vi "ATF Storage-DO_Write.vi"(7 "Period":i64=100, 8 "error in (no error)":errorcluster, 10 "Data FIFO Ref":T1, 11 "Refnum in":refnum<k21>) -> (0 "error out":errorcluster, 3 "Refnum out":refnum<k21>)   [LabVIEW 2022 SP3]
uses:
  RT Controls/ATF Storage-Data FIFO.ctl
  <vilib>/Platform/TimedLoop/XDataNode/timing_clust.ctl
  <vilib>/Platform/TimedLoop/XDataNode/nitl_modes.ctl
  <vilib>/Platform/TimedLoop/XDataNode/wakeup.ctl
  RT Controls/ATF Storage Haelth.ctl
  <vilib>/DAQmx/write.llb/DAQmx Write (Digital 1D Bool NChan 1Samp 1Line).vi
  RT Support/ATF Storage-RT_Global_R.vi
  <vilib>/DAQmx/miscellaneous.llb/DAQmx Fill In Error Info.vi
  <vilib>/platform/TimedLoop/XDataNode/XDataNode.xnode
  <vilib>/Platform/TimedLoop/XDataNode/XDNodeRunTimeDep.lvlib
panel:
  out "overflow?":bool
  out "x":u32
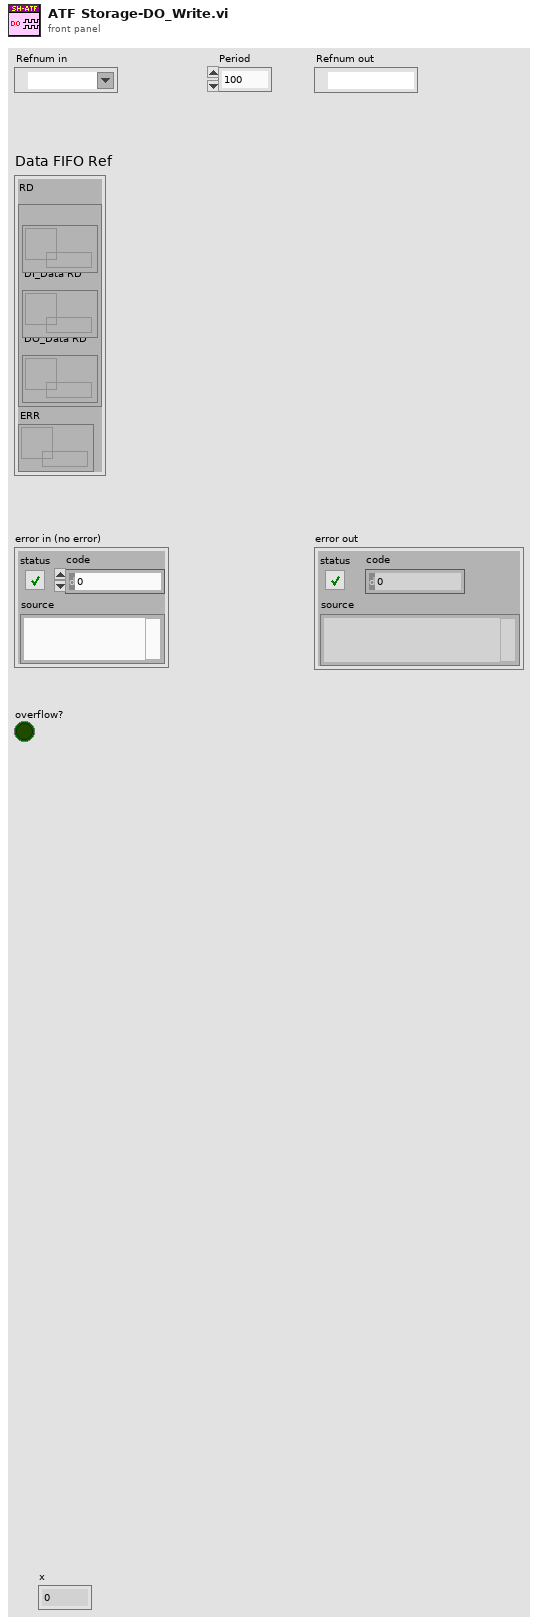
[diagram p1: front panel]
types:
  T1 = typedef "ATF Storage-Data FIFO.ctl" = cluster{"RD":cluster{"AI_V_Data RD":refnum<queue>, "DI_Data RD":refnum<queue>, "DO_Data RD":refnum<queue>}, "ERR":refnum<queue>}
  T2 = enum16{"Init", "Read", "Write 'All'", "Write 'n'", "Write Safe Value", "Write Start Time", "Overwrite Pattern", "Overwrite Pattern with Start", "Append Pattern", "Start Pattern Mode", "Abort Pattern Mode", "Read 1"}
  T3 = typedef "XDNodeRunTimeDep.lvlib/timing_clust.ctl" = cluster{"Expected End [f-1]":u64, "Actual End [f-1]":u64, "Finished Late? [f-1]":bool, "Expected End [i-1]":u64, "Actual End [i-1]":u64, "Finished Late? [i-1]":bool, "Expected Start [i]":u64, "Actual Start [i]":u64, "Expected Start [f]":u64, "Actual Start [f]":u64, "Source Name":string, "Structure Name":string, "Period":i64, "Deadline":i64, "Offset":i64, "Start":i64, "Priority":i32, "Timeout":i32, "Mode":T4, "Wakeup Reason":T5, "Error":errorcluster, "Source Type":string, "Secondary Source Type":string, "Global End Time":u64, "Global Start Time":u64, "Frame Duration":u64, "Iteration Duration":u64, "Assigned CPU":i32, "I/O Scan Engine Mode":u32}
  T4 = typedef "XDNodeRunTimeDep.lvlib/nitl_modes.ctl" = enum32{"No Change", "Process missed periods, maintain original phase", "Discard missed periods, maintain original phase", "Process missed periods, ignore original phase", "Discard missed periods, ignore original phase"}
  T5 = typedef "XDNodeRunTimeDep.lvlib/wakeup.ctl" = enum32{"Normal", "Aborted", "Asynchronous wakeup", "Timing source error", "Timed loop error", "Timeout"}
  T6 = typedef "ATF Storage Haelth.ctl" = enum16{"AI C", "AI V", "AO", "DI", "DO", "TC", "ACC", "RT Str", "DR A"}
  T7 = enum16{"Init", "Read 'All'", "Read 'n'", "Read '1'", "Write '1'", "Write 'n'", "Write 'All'"}
  T8 = cluster{"Start DAQ":bool, "Stop DAQ":bool, "RT Stop":bool, "RT Exit":bool, "Start Seq":bool}
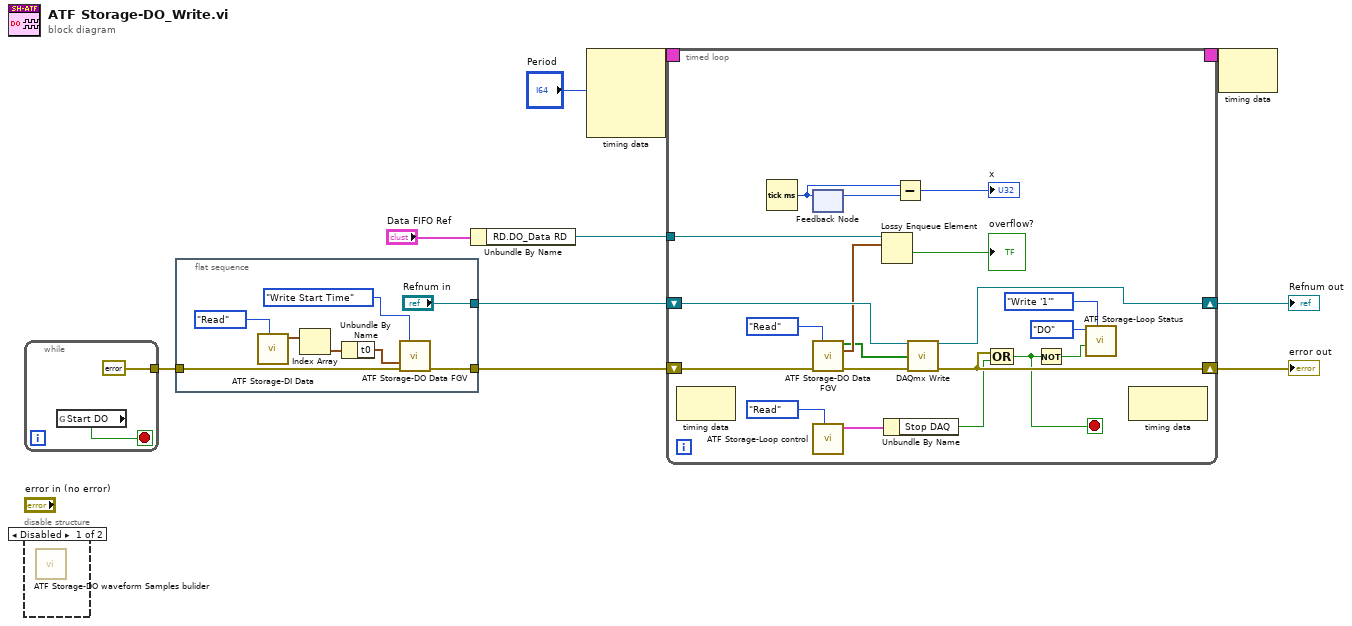
[diagram p0: block diagram]
diagram:
  n1 = while {
    tunnel: [errorcluster {"status"=FALSE, "code"=0, "source"=""} ("error in (no error)")] -> w4
    stop <- w12 stop-if-true
    n2 = global read "ATF Storage-RT_Global_R.vi" "Start DO"() -> (w12:bool)
  }
  n3 = disable-structure shown="Disabled" {
    frame Disabled {
      n4 = call "ATF Storage-DO waveform Samples bulider.vi"() -> ()  [unwired: 12 in]
    }
    frame Enabled {
    }
  }
  n5 = flat-sequence {
    tunnel: w4 -> [w18]
    tunnel: ["Refnum in"] -> w6
    tunnel: [w19] -> w5
    frame #0 {
      n6 = call "ATF Storage-DI Data.vi"("Enum"=enum16{"Write", "Read"}."Read") -> ("Out_DI data"=w17:digitalwaveform[])  [unwired: 10 in]
      n7 = Index Array(array=w17) -> (element=w16:digitalwaveform)  [unwired: 1 in]
      n8 = Unbundle By Name(w16) -> ("t0"=w14:timestamp)
      n9 = call "ATF Storage-DO Data FGV.vi"("Option"=T2."Write Start Time", "Time Stamp In"=w14, "error in (no error)"=w18) -> ("error out"=w19:errorcluster)  [unwired: 6 in, 6 out]
    }
  }
  n10 = Unbundle By Name("Data FIFO Ref") -> ("RD.DO_Data RD"=w7:refnum<queue>)
  n11 = node-c288("Period") -> (w3:T3)  [unwired: 3 in]
  n12 = timed-loop {
    tunnel: w7 -> [w37]
    shift-right: [w38] -> w9
    shift-left: w6 -> [w40]
    shift-right: [w39] -> w10
    shift-left: w5 -> [w30]
    timing: w3 -> [_]
    timing-out: [_] -> w2
    stop <- w21 stop-if-true
    n13 = node-c288() -> ()  [unwired: 1 in, 1 out]
    n14 = Tick Count (ms)() -> (millisecond timer value=w36:u32)
    n15 = feedback #1() -> (w35:u32)  [unwired: 1 in]
    n16 = feedback-in #1(w36) -> ()
    n17 = call "ATF Storage-DO Data FGV.vi"("Option"=T2."Read", "error in (no error)"=w30) -> ("DO Values Out"=w27:bool[], "All data out"=w28:waveform(dbl)[], "error out"=w29:errorcluster)  [unwired: 7 in, 4 out]
    n18 = call "ATF Storage-Loop control.vi"("Action"=enum16{"Init", "Write", "Read"}."Read") -> ("Loop Control out"=w33:T8)  [unwired: 9 in, 1 out]
    n19 = Lossy Enqueue Element(queue=w37, element=w28) -> (overflow?=→"overflow?":bool)  [unwired: 1 in, 3 out]
    n20 = Unbundle By Name(w33) -> ("Stop DAQ"=w31:bool)
    n21 = Subtract(x=w36, y=w35) -> (x-y=→"x":u32)
    n22 = call-poly <vilib>:"DAQmx Write.vi"("task/channels in"=w40, "data"=w27, "error in"=w29) -> ("task out"=w38:refnum<k21>, "error out"=w39:errorcluster)  [unwired: 10 in, 1 out]
    n23 = Compound Arithmetic op=OR(w39, w31) -> (w21:bool)
    n24 = Not(x=w21) -> (.not. x?=w23:bool)
    n25 = call "ATF Storage-Loop Status.vi"("Option"=T7."Write '1'", "Status"=w23, "Loop"=ATF_Storage_Haelth."DO") -> ()  [unwired: 6 in, 3 out]
    n26 = node-c288() -> ()  [unwired: 1 in, 1 out]
  }
  "Refnum out" <- w9
  "error out" <- w10
  n27 = node-c288(w2) -> ()  [unwired: 1 out]
